vi "QPen.vi"(4 "capStyle (SquareCap)":T2=16 items=["FlatCap"=0, "SquareCap"=16, "RoundCap"=32, "MPenCapStyle"=48], 6 "style (SolidLine)":T3=1 items=["NoPen"=0, "SolidLine"=1, "DashLine"=2, "DotLine"=3, "DashDotLine"=4, "DashDotDotLine"=5, "CustomDashLine"=6, "MPenStyle"=15], 7 "joinStyle (BevelJoin)":T1=64 items=["MiterJoin"=0, "BevelJoin"=64, "RoundJoin"=128, "SvgMiterJoin"=256, "MPenJoinStyle"=448], 8 "Error In":errorcluster, 9 "width (0)":dbl, 10 "brush":u32(colorbox)) -> (0 "Error Out":errorcluster, 3 "New QPen":refnum<class "QPen.lvclass">)   [LabVIEW 2014, in "QPen.lvclass"]
doc: "LabVIEW-specific documentation is not yet available. See <b>https://doc.qt.io/qt-5/qpen.html#QPen</b>"
uses:
  QPen.lvclass
  LQ Core/Qt/PenStyle.ctl
  LQ Core/Qt/PenCapStyle.ctl
  LQ Core/Qt/PenJoinStyle.ctl
  LQ Core/LQSerialData/LQSerialData.lvclass/LQSerialData.ctl
  LQ Core/LQ Core.lvlib
  LQ Core/LQSerialData/LQSerialData.lvclass
  LQ Core/Qt/Qt.lvlib
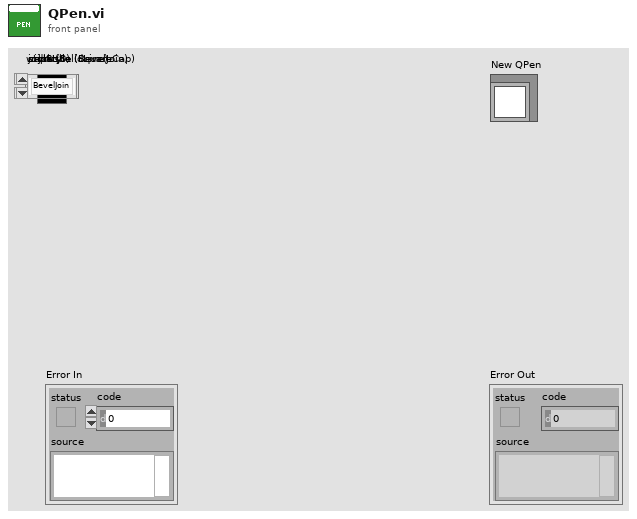
[diagram p1: front panel]
types:
  T1 = typedef "Qt.lvlib/PenJoinStyle.ctl" = i32
  T2 = typedef "Qt.lvlib/PenCapStyle.ctl" = i32
  T3 = typedef "Qt.lvlib/PenStyle.ctl" = i32
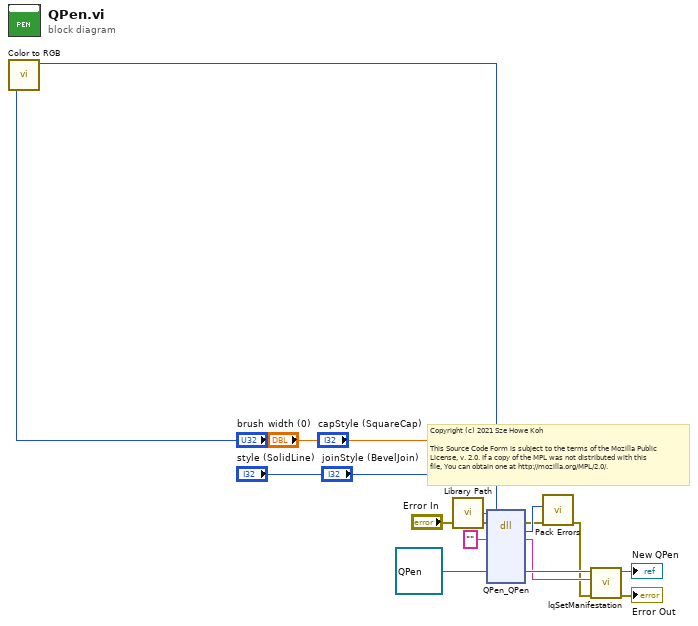
[diagram p0: block diagram]
diagram:
  # "Copyright (c) 2021 Sze Howe Koh\n\nThis Source Code Form is subject to the terms of the Mozilla Public\nLicense, v. 2.0. If a copy of the MPL was not distributed with this\nfile, You can obtain one at http://mozilla.org/MPL/2.0/."
  n1 = call <vilib>:"Color to RGB.vi"("Color"="brush") -> ("Resolved Color"=w5:u32)  [unwired: 3 out]
  n2 = call "Library Path.vi"() -> ("Library Path"=w11:path)
  n3 = dll-call lib="?" fn="QPen_QPen"(path in=w11, error in="Error In", "_retVal"="", "brush"=w5, "width"="width (0)", "style"="style (SolidLine)", "capStyle"="capStyle (SquareCap)", "joinStyle"="joinStyle (BevelJoin)") -> (error out=w9:errorcluster, w10:i32, "_retVal"=w12:string)  [unwired: 6 in, 1 out]
  n4 = call "Pack Errors.vi"("Error In"=w9, "Error Code"=w10) -> ("Error Out"=w8:errorcluster)  [unwired: 9 in]
  n5 = call "lqSetManifestation.vi"("Error In"=w8, "Manifestation"=w12, "LQSerialData in"=refnum<class "QPen.lvclass"> refnum ("QPen")) -> ("Error Out"=→"Error Out":errorcluster, "LQSerialData out"=→"New QPen":refnum<class "QPen.lvclass">)  [unwired: 7 in]
